vi "Main.vi"(8 "error in":errorcluster, 11 "Host NI 9205 Demo in":refnum<class "Host NI 9205 Demo.lvclass">) -> (0 "error out":errorcluster, 3 "Host NI 9205 Demo out":refnum<class "Host NI 9205 Demo.lvclass">)   [LabVIEW 2017, in "Host NI 9205 Demo.lvclass"]
doc: "The <b>Queued Message Handler</b> of the Worker that owns this VI."
uses:
  Host NI 9205 Demo.lvclass
  C:/Program Files (x86)/National Instruments/LabVIEW 2017/vi.lib/addons/_Workers/Library/Classes/Worker/Worker.lvclass
  Host NI 9205 Demo.lvclass/Host NI 9205 Demo.ctl
  Initialization Data.ctl
  Response Cases.ctl
  Main UI/rqp_Embed System Monitor UI.ctl
  Main UI/rqp_TCP Client Connection Notify.ctl
  Shared/TCP Data Format.ctl
  Shared/TCP Data KEYS.ctl
  Main UI/rqp_TCP Client Incoming Data.ctl
  System Monitor UI/rqp_Update cRIO System Data.ctl
  TCP Server/TCP Server/rqp_Start Listening.ctl
  <vilib>/addons/_Workers/Library/Classes/Message Queue/Message Queue.lvclass
  System Monitor UI/System Monitor UI.lvclass
  Main UI/Main UI.lvclass
  TCP Server/TCP Server/TCP Server.lvclass
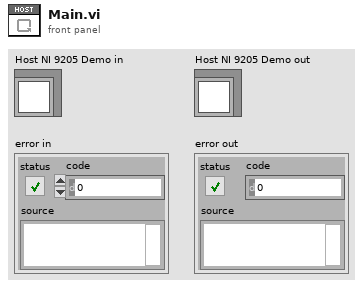
[diagram p1: front panel]
types:
  T1 = typedef "Host NI 9205 Demo.lvclass/Initialization Data.ctl" = cluster{"Response Cases":T2}
  T2 = typedef "Host NI 9205 Demo.lvclass/Response Cases.ctl" = cluster{"Placeholder - Can be deleted":string}
  T3 = typedef "Main UI.lvclass/rqp_Embed System Monitor UI.ctl" = cluster{"Main VI Ref":refnum<vi>}
  T4 = typedef "Main UI.lvclass/rqp_TCP Client Connection Notify.ctl" = cluster{"Client Name":string, "IP Address":string, "Connected?":bool}
  T5 = typedef "TCP Data Format.ctl" = cluster{"KEY":T6, "Data":string}
  T6 = typedef "TCP Data KEYS.ctl" = enum16{"RT System Monitor", "FPGA Data"}
  T7 = typedef "Main UI.lvclass/rqp_TCP Client Incoming Data.ctl" = cluster{"Data as String":string}
  T8 = typedef "System Monitor UI.lvclass/rqp_Update cRIO System Data.ctl" = cluster{"Data as String":string}
  T9 = typedef "TCP Server.lvlib/TCP Server.lvclass/rqp_Start Listening.ctl" = cluster{"Server Name":string, "Server IP Address":string, "Server Port":u16}
  T10 = typedef "System Monitor UI.lvclass/rwr_Get Main VI Ref Reply.ctl" = cluster{"Main VI Ref":refnum<vi>}
  T11 = typedef "TCP Server.lvlib/TCP Server.lvclass/rsp_Connection Notify.ctl" = cluster{"Client Name":string, "IP Address":string, "Connected?":bool}
  T12 = typedef "TCP Server.lvlib/TCP Server.lvclass/rsp_Incoming Data.ctl" = cluster{"Client Name":string, "Data":string}
  T13 = typedef "Main UI.lvclass/rsp_TCP Server Start Listening.ctl" = cluster{"Server Name":string, "Server Port":u16}
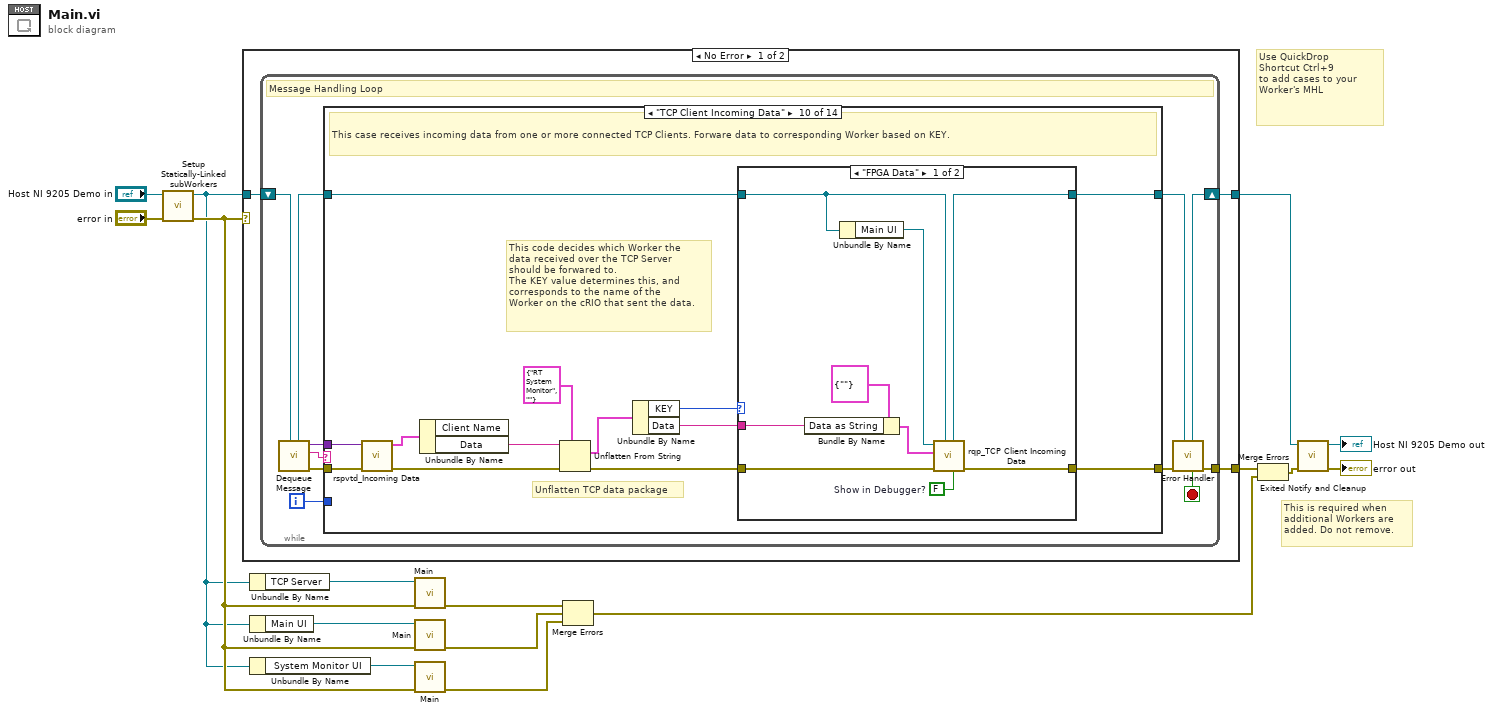
[diagram p0: block diagram]
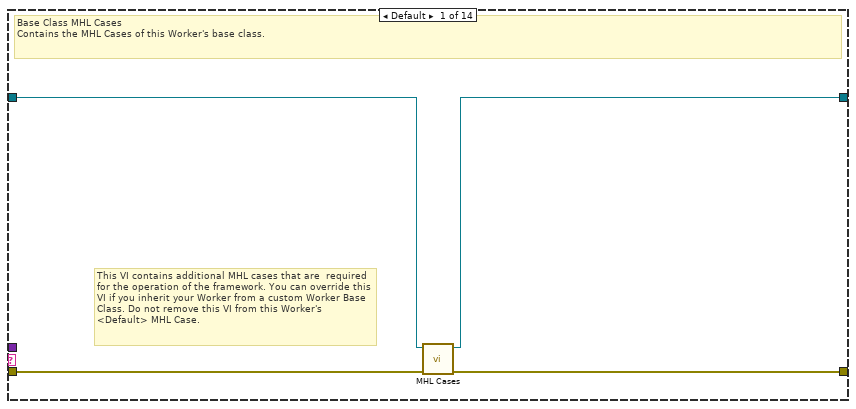
[diagram p2: hidden frame]
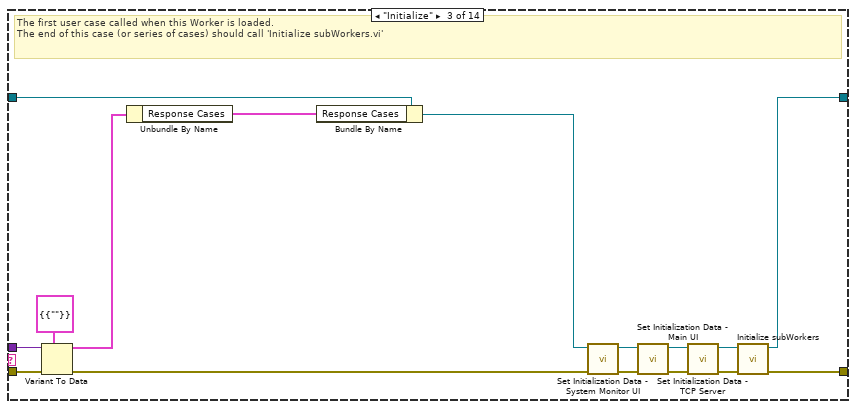
[diagram p4: hidden frame]
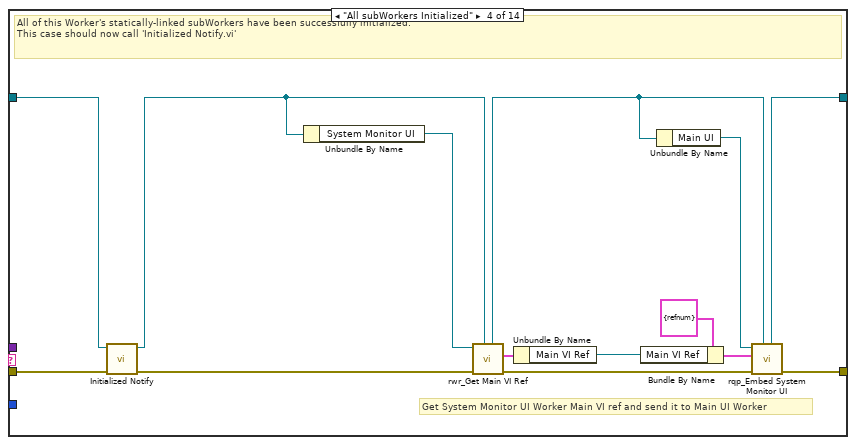
[diagram p5: hidden frame]
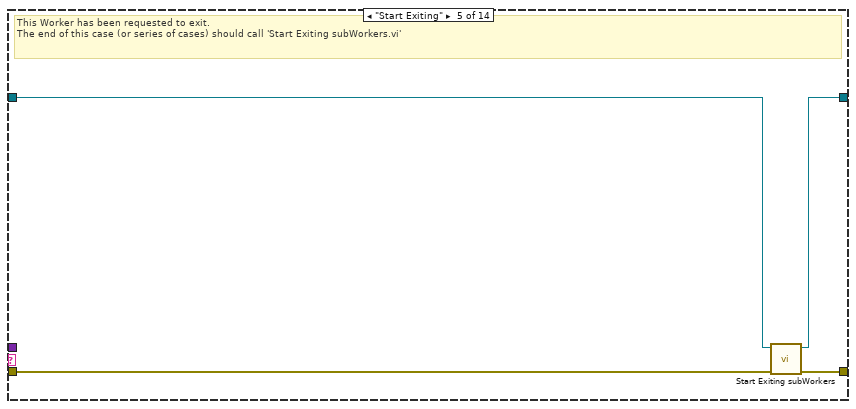
[diagram p6: hidden frame]
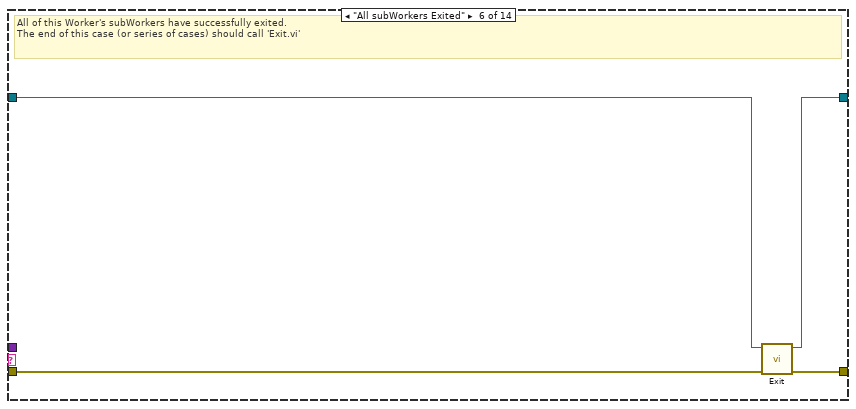
[diagram p7: hidden frame]
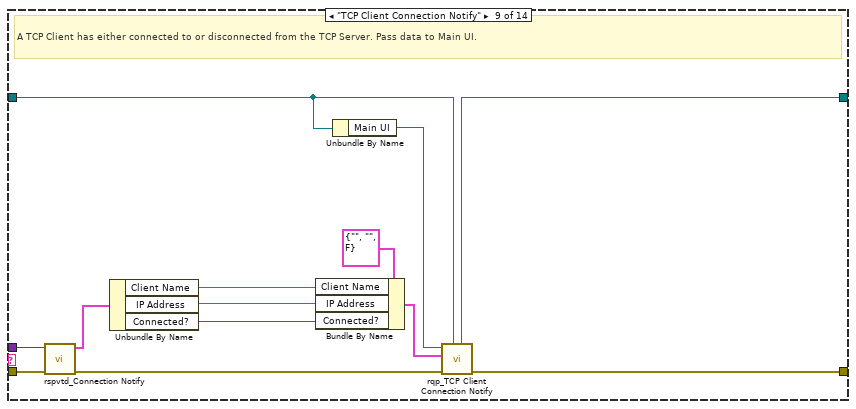
[diagram p10: hidden frame]
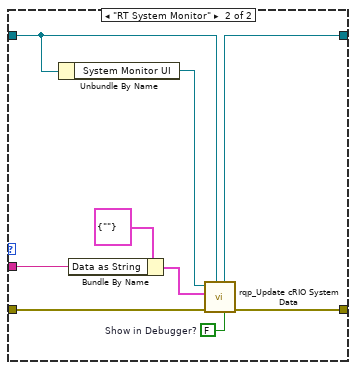
[diagram p11: hidden frame]
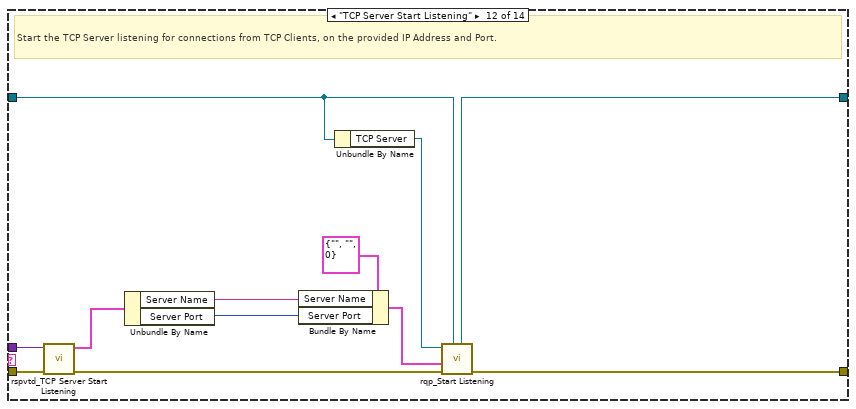
[diagram p13: hidden frame]
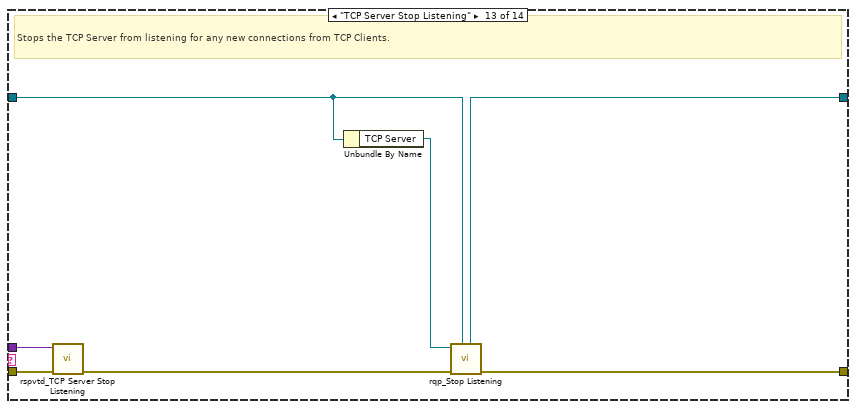
[diagram p14: hidden frame]
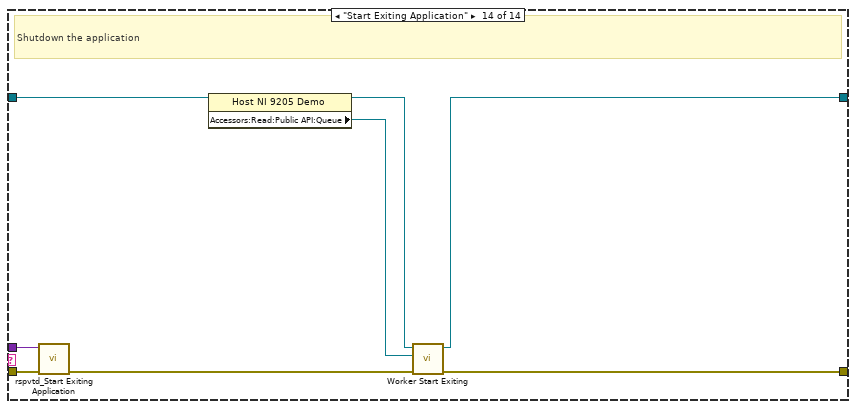
[diagram p15: hidden frame]
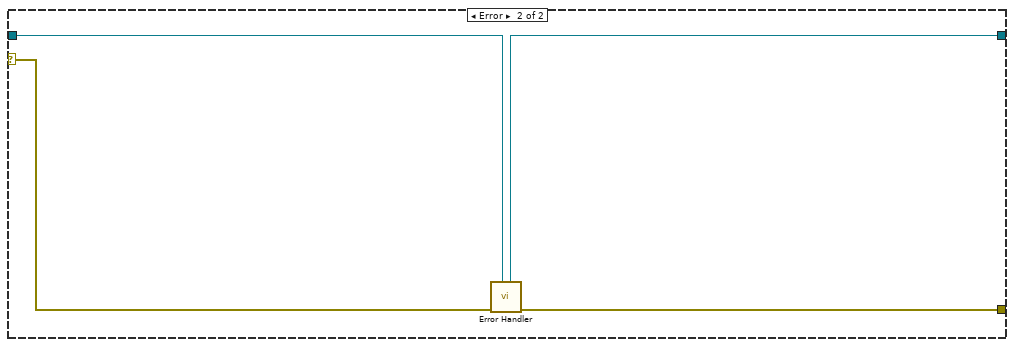
[diagram p16: hidden frame]
diagram:
  # "Use QuickDrop\nShortcut Ctrl+9\nto add cases to your\nWorker's MHL"
  # "This is required when additional Workers are added. Do not remove."
  n1 = call "Setup Statically-Linked subWorkers.vi"("error in"="error in", "Host NI 9205 Demo in"="Host NI 9205 Demo in") -> ("error out"=w10:errorcluster, "Host NI 9205 Demo out"=w8:refnum<class "Host NI 9205 Demo.lvclass">)  [unwired: 8 in]
  n2 = case shown="No Error" w10 {
    tunnel: w8 -> [w17 w153]
    tunnel: [w19 w154] -> w15
    tunnel: [w18 w152] -> w16
    selector: w10 -> [_ w155]
    frame No Error {
      n3 = while {
        shift-right: [w28] -> w18
        shift-left: w17 -> [w30]
        tunnel: [w29] -> w19
        i -> [w20]
        stop <- w21 stop-if-true
        # "Message Handling Loop"
        n4 = call-dynamic "Dequeue Message.vi"("Worker"=w30) -> ("error out"=w27:errorcluster, "Case out"=w22:string, "Data out"=w23:variant, "Worker out"=w25:refnum<class "Host NI 9205 Demo.lvclass">)  [unwired: 6 in, 1 out]
        n5 = case "Worker MHL Case Structure (DO NOT CHANGE LABEL NAME)" shown="\"TCP Client Incoming Data\"" w22 {
          tunnel: w27 -> [w34 w35 w50 w66 w67 w74 w76 w78 w90 w103 w124 w136 w140 w151]
          tunnel: [w33 w35 w52 w59 w70 w73 w76 w78 w87 w101 w124 w133 w139 w150] -> w26
          tunnel: w25 -> [w32 w36 w49 w64 w68 w72 w75 w77 w85 w99 w123 w131 w137 w149]
          tunnel: [w31 w36 w51 w58 w69 w71 w75 w77 w86 w100 w123 w132 w138 w148] -> w24
          tunnel: w23 -> [_ _ w47 _ _ _ _ _ w89 w104 _ w134 w141 w144]
          tunnel: w20 -> [_ _ _ _ _ _ _ _ _ _ _ _ _ _]
          frame Default {
            # "This VI contains additional MHL cases that are  required for the operation of the framework. You can override this VI if you inherit your Worker from a custom Worker Base Class. Do not remove this VI from this Worker's <Default> MHL Case."
            # "Base Class MHL Cases\nContains the MHL Cases of this Worker's base class."
            n6 = call-dynamic "MHL Cases.vi"("error in"=w34, "Worker in"=w32) -> ("error out"=w33:errorcluster, "Worker out"=w31:refnum<class "Host NI 9205 Demo.lvclass">)  [unwired: 8 in]
          }
          frame "------------ FRAMEWORK CASES -----------" {
            # "Start of Workers Framework Cases"
          }
          frame "Initialize" {
            # "The first user case called when this Worker is loaded.\nThe end of this case (or series of cases) should call 'Initialize subWorkers.vi'"
            n7 = Variant To Data(error in=w50, type=T1 {"Response Cases"={"Placeholder - Can be deleted"=""}} ("Cluster"), Variant=w47) -> (data=w46:T1, error out=w48:errorcluster)
            n8 = Unbundle By Name(w46) -> ("Response Cases"=w45:T2)
            n9 = Bundle By Name(cluster=w49, "Response Cases"=w45) -> (w38:refnum<class "Host NI 9205 Demo.lvclass">)
            n10 = call "Set Initialization Data - System Monitor UI.vi"("error in"=w48, "Host NI 9205 Demo in"=w38) -> ("error out"=w39:errorcluster, "Host NI 9205 Demo out"=w37:refnum<class "Host NI 9205 Demo.lvclass">)  [unwired: 8 in]
            n11 = call "Set Initialization Data - Main UI.vi"("error in"=w39, "Host NI 9205 Demo in"=w37) -> ("error out"=w41:errorcluster, "Host NI 9205 Demo out"=w40:refnum<class "Host NI 9205 Demo.lvclass">)  [unwired: 8 in]
            n12 = call "Set Initialization Data - TCP Server.vi"("error in"=w41, "Host NI 9205 Demo in"=w40) -> ("error out"=w43:errorcluster, "Host NI 9205 Demo out"=w42:refnum<class "Host NI 9205 Demo.lvclass">)  [unwired: 8 in]
            n13 = call-dynamic "Initialize subWorkers.vi"("error in"=w43, "Worker"=w42) -> ("error out"=w52:errorcluster, "dup Worker out"=w51:refnum<class "Host NI 9205 Demo.lvclass">)  [unwired: 8 in]
          }
          frame "All subWorkers Initialized" {
            # "Get System Monitor UI Worker Main VI ref and send it to Main UI Worker"
            # "All of this Worker's statically-linked subWorkers have been successfully initialized.\nThis case should now call 'Initialized Notify.vi'"
            n14 = call-dynamic "Initialized Notify.vi"("error in"=w66, "Worker"=w64) -> ("error out"=w65:errorcluster, "dup Worker out"=w62:refnum<class "Host NI 9205 Demo.lvclass">)  [unwired: 8 in]
            n15 = Unbundle By Name(w62) -> ("System Monitor UI"=w61:refnum<class "System Monitor UI.lvclass">)
            n16 = call "rwr_Get Main VI Ref.vi"("Caller in"=w62, "error in"=w65, "System Monitor UI in"=w61) -> ("error out"=w63:errorcluster, "Reply Data out"=w60:T10, "dup Caller out"=w57:refnum<class "Host NI 9205 Demo.lvclass">)  [unwired: 5 in, 1 out]
            n17 = Unbundle By Name(w60) -> ("Main VI Ref"=w53:refnum<vi>)
            n18 = Bundle By Name(cluster=T3 {"Main VI Ref"=refnum} ("Data in"), "Main VI Ref"=w53) -> (w54:T3)
            n19 = Unbundle By Name(w57) -> ("Main UI"=w56:refnum<class "Main UI.lvclass">)
            n20 = call "rqp_Embed System Monitor UI.vi"("Caller in"=w57, "error in"=w63, "Data in"=w54, "Main UI in"=w56) -> ("error out"=w59:errorcluster, "dup Caller out"=w58:refnum<class "Host NI 9205 Demo.lvclass">)  [unwired: 5 in, 1 out]
          }
          frame "Start Exiting" {
            # "This Worker has been requested to exit. \nThe end of this case (or series of cases) should call 'Start Exiting subWorkers.vi'"
            n21 = call-dynamic "Start Exiting subWorkers.vi"("error_in"=w67, "Worker"=w68) -> ("error out"=w70:errorcluster, "dup Worker out"=w69:refnum<class "Host NI 9205 Demo.lvclass">)  [unwired: 8 in]
          }
          frame "All subWorkers Exited" {
            # "All of this Worker's subWorkers have successfully exited. \nThe end of this case (or series of cases) should call 'Exit.vi'"
            n22 = call-dynamic "Exit.vi"("error_in"=w74, "Worker"=w72) -> ("error out"=w73:errorcluster, "dup Worker out"=w71:refnum<class "Host NI 9205 Demo.lvclass">)  [unwired: 8 in]
          }
          frame "------------- RESPONSE CASES --------------" {
            # "Start of Workers Response Cases"
          }
          frame "~~~~~~~~~~ TCP Server ~~~~~~~~~~" {
            # "TCP Server Registered Responses"
          }
          frame "TCP Client Connection Notify" {
            # "A TCP Client has either connected to or disconnected from the TCP Server. Pass data to Main UI."
            n23 = call "rspvtd_Connection Notify.vi"("error in"=w90, "Data in"=w89) -> ("error out"=w88:errorcluster, "Data out"=w91:T11)  [unwired: 8 in]
            n24 = Unbundle By Name(w91) -> ("Client Name"=w81:string, "IP Address"=w80:string, "Connected?"=w79:bool)
            n25 = Bundle By Name(cluster=T4 {"Client Name"="", "IP Address"="", "Connected?"=FALSE} ("Data in"), "Client Name"=w81, "IP Address"=w80, "Connected?"=w79) -> (w82:T4)
            n26 = Unbundle By Name(w85) -> ("Main UI"=w84:refnum<class "Main UI.lvclass">)
            n27 = call "rqp_TCP Client Connection Notify.vi"("Caller in"=w85, "error in"=w88, "Data in"=w82, "Main UI in"=w84) -> ("error out"=w87:errorcluster, "dup Caller out"=w86:refnum<class "Host NI 9205 Demo.lvclass">)  [unwired: 5 in, 1 out]
          }
          frame "TCP Client Incoming Data" {
            # "Unflatten TCP data package"
            # "This code decides which Worker the \ndata received over the TCP Server\nshould be forwared to.\nThe KEY value determines this, and\ncorresponds to the name of the\nWorker on the cRIO that sent the data."
            # "This case receives incoming data from one or more connected TCP Clients. Forware data to corresponding Worker based on KEY."
            n28 = call "rspvtd_Incoming Data.vi"("error in"=w103, "Data in"=w104) -> ("error out"=w102:errorcluster, "Data out"=w98:T12)  [unwired: 8 in]
            n29 = Unbundle By Name(w98) -> ("Data"=w96:string)  [unwired: 1 out]
            n30 = Unflatten From String(type=T5 {"KEY"=enum."RT System Monitor", "Data"=""} ("Data in"), binary string=w96, error in (no error)=w102) -> (value=w94:T5, error out=w97:errorcluster)  [unwired: 2 in, 1 out]
            n31 = Unbundle By Name(w94) -> ("KEY"=w92:T6, "Data"=w93:string)
            n32 = case shown="\"FPGA Data\"" w92 {
              tunnel: [w113 w122] -> w101
              tunnel: [w112 w121] -> w100
              tunnel: w99 -> [w110 w119]
              tunnel: w97 -> [w106 w115]
              tunnel: w93 -> [w105 w114]
              frame "FPGA Data" {
                w107 = FALSE  # Show in Debugger?
                n33 = Bundle By Name(cluster=T7 {"Data as String"=""} ("Data in"), "Data as String"=w105) -> (w108:T7)
                n34 = Unbundle By Name(w110) -> ("Main UI"=w111:refnum<class "Main UI.lvclass">)
                n35 = call "rqp_TCP Client Incoming Data.vi"("Show in Debugger?"=w107, "Caller in"=w110, "error in"=w106, "Data in"=w108, "Main UI in"=w111) -> ("error out"=w113:errorcluster, "dup Caller out"=w112:refnum<class "Host NI 9205 Demo.lvclass">)  [unwired: 4 in, 1 out]
              }
              frame "RT System Monitor" {
                w116 = FALSE  # Show in Debugger?
                n36 = Unbundle By Name(w119) -> ("System Monitor UI"=w120:refnum<class "System Monitor UI.lvclass">)
                n37 = Bundle By Name(cluster=T8 {"Data as String"=""} ("Data in"), "Data as String"=w114) -> (w117:T8)
                n38 = call "rqp_Update cRIO System Data.vi"("Show in Debugger?"=w116, "Caller in"=w119, "error in"=w115, "Data in"=w117, "System Monitor UI in"=w120) -> ("error out"=w122:errorcluster, "dup Caller out"=w121:refnum<class "Host NI 9205 Demo.lvclass">)  [unwired: 4 in, 1 out]
              }
            }
          }
          frame "~~~~~~~~~~ Main UI ~~~~~~~~~~" {
            # "Main UI Registered Responses"
          }
          frame "TCP Server Start Listening" {
            # "Start the TCP Server listening for connections from TCP Clients, on the provided IP Address and Port."
            n39 = call "rspvtd_TCP Server Start Listening.vi"("error in"=w136, "Data in"=w134) -> ("error out"=w135:errorcluster, "Data out"=w127:T13)  [unwired: 8 in]
            n40 = Unbundle By Name(w127) -> ("Server Name"=w126:string, "Server Port"=w125:u16)
            n41 = Bundle By Name(cluster=T9 {"Server Name"="", "Server IP Address"="", "Server Port"=0} ("Data in"), "Server Name"=w126, "Server Port"=w125) -> (w128:T9)
            n42 = Unbundle By Name(w131) -> ("TCP Server"=w130:refnum<class "TCP Server.lvclass">)
            n43 = call "rqp_Start Listening.vi"("Caller in"=w131, "error in"=w135, "Data in"=w128, "TCP Server in"=w130) -> ("error out"=w133:errorcluster, "dup Caller out"=w132:refnum<class "Host NI 9205 Demo.lvclass">)  [unwired: 5 in, 1 out]
          }
          frame "TCP Server Stop Listening" {
            # "Stops the TCP Server from listening for any new connections from TCP Clients."
            n44 = call "rspvtd_TCP Server Stop Listening.vi"("error in"=w140, "Data in"=w141) -> ("error out"=w143:errorcluster)  [unwired: 8 in, 1 out]
            n45 = Unbundle By Name(w137) -> ("TCP Server"=w142:refnum<class "TCP Server.lvclass">)
            n46 = call "rqp_Stop Listening.vi"("Caller in"=w137, "error in"=w143, "TCP Server in"=w142) -> ("error out"=w139:errorcluster, "dup Caller out"=w138:refnum<class "Host NI 9205 Demo.lvclass">)  [unwired: 6 in, 1 out]
          }
          frame "Start Exiting Application" {
            # "Shutdown the application"
            n47 = call "rspvtd_Start Exiting Application.vi"("error in"=w151, "Data in"=w144) -> ("error out"=w145:errorcluster)  [unwired: 8 in, 1 out]
            n48 = property class="Host NI 9205 Demo"(reference=w149) -> (reference out=w147:refnum<class "Host NI 9205 Demo.lvclass">, "Accessors:Read:Public API:Queue"=w146:refnum<class "Message Queue.lvclass">)  [unwired: 1 in, 1 out]
            n49 = call-dynamic "Worker Start Exiting.vi"("error_in"=w145, "Message Queue"=w146, "Worker"=w147) -> ("error out"=w150:errorcluster, "dup Worker out"=w148:refnum<class "Host NI 9205 Demo.lvclass">)  [unwired: 7 in]
          }
        }
        n50 = call-dynamic "Error Handler.vi"("Worker"=w24, "error_in"=w26) -> ("error out"=w29:errorcluster, "Stop Loop"=w21:bool, "Worker out"=w28:refnum<class "Host NI 9205 Demo.lvclass">)  [unwired: 7 in]
      }
    }
    frame Error {
      n51 = call-dynamic "Error Handler.vi"("Worker"=w153, "error_in"=w155) -> ("error out"=w154:errorcluster, "Worker out"=w152:refnum<class "Host NI 9205 Demo.lvclass">)  [unwired: 7 in, 1 out]
    }
  }
  n52 = Unbundle By Name(w8) -> ("TCP Server"=w5:refnum<class "TCP Server.lvclass">)
  n53 = Unbundle By Name(w8) -> ("Main UI"=w3:refnum<class "Main UI.lvclass">)
  n54 = Unbundle By Name(w8) -> ("System Monitor UI"=w1:refnum<class "System Monitor UI.lvclass">)
  n55 = call-dynamic "Main.vi"("error in"=w10, "TCP Server in"=w5) -> ("error out"=w7:errorcluster)  [unwired: 8 in, 1 out]
  n56 = call-dynamic "Main.vi"("error in"=w10, "Main UI in"=w3) -> ("error out"=w4:errorcluster)  [unwired: 8 in, 1 out]
  n57 = call-dynamic "Main.vi"("error in"=w10, "System Monitor UI in"=w1) -> ("error out"=w2:errorcluster)  [unwired: 8 in, 1 out]
  n58 = Merge Errors(w7, w4, w2) -> (w6:errorcluster)
  n59 = Merge Errors(w15, w6) -> (w12:errorcluster)
  n60 = call-dynamic "Exited Notify and Cleanup.vi"("error_in"=w12, "Worker"=w16) -> ("error out"=→"error out":errorcluster, "dup Worker out"=→"Host NI 9205 Demo out":refnum<class "Host NI 9205 Demo.lvclass">)  [unwired: 8 in]
